vi "数据记录.vi"(11 "写入字段":string) -> (3 "连接的字符串":string)   [LabVIEW 2016, in "数据传输系统.lvlib"]
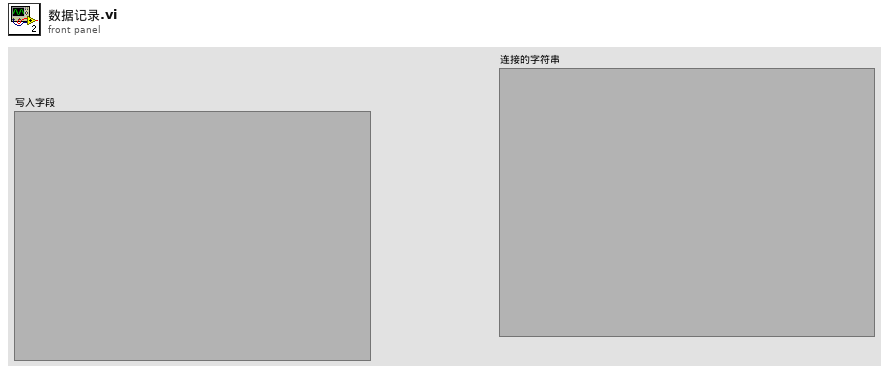
[diagram p1: front panel]
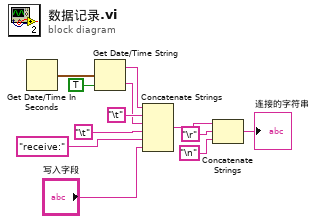
[diagram p0: block diagram]
diagram:
  n1 = Get Date/Time In Seconds() -> (seconds since 1Jan1904=w4:timestamp)
  n2 = Get Date/Time String(seconds (now)=w4, want seconds? (F)=TRUE ("需要秒？(F)")) -> (date string=w7:string, time string=w5:string)  [unwired: 1 in]
  n3 = Concatenate Strings(w7, "\t", w5, "\t", "receive:" ("字符串"), "写入字段") -> (w3:string)
  n4 = Concatenate Strings(w3, "\r", "\n") -> (→"连接的字符串":string)
